vi "Configure Dialog.vi"(8 "error in (no error)":errorcluster, 11 "Initiate Acquisition Msg in":refnum<class "Initiate Acquisition Msg.lvclass">) -> (0 "error out":errorcluster, 2 "Ok?":bool, 3 "Initiate Acquisition Msg out":refnum<class "Initiate Acquisition Msg.lvclass">)   [LabVIEW 2014, in "CS++Scope.lvlib" / "Initiate Acquisition Msg.lvclass"]
uses:
  Initiate Acquisition Msg.lvclass
  Initiate Acquisition Msg.lvclass/Initiate Acquisition Msg.ctl
panel:
  in  "OK Button":bool
  in  "Cancel Button":bool
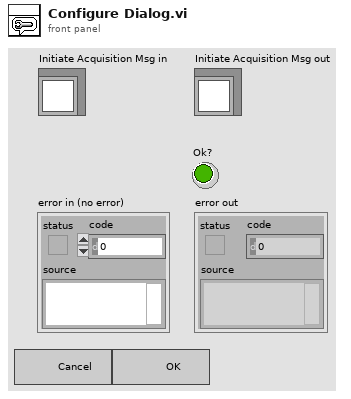
[diagram p1: front panel]
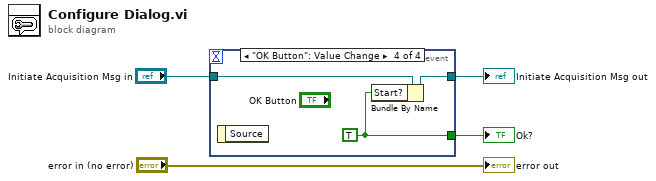
[diagram p0: block diagram]
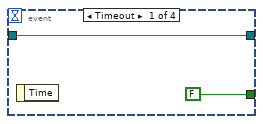
[diagram p2: hidden frame]
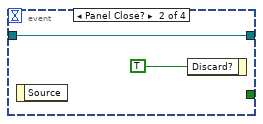
[diagram p3: hidden frame]
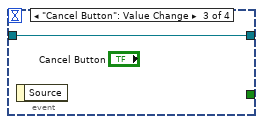
[diagram p4: hidden frame]
diagram:
  n1 = event shown="[3] \"OK Button\": Value Change" {
    selector: _ -> [_ _ _ _]
    dyn-events: _ -> [_ _ _ _]
    timeout: _ -> [_ _ _ _]
    tunnel: [w6 w7 w9 w11] -> w3
    tunnel: "Initiate Acquisition Msg in" -> [w6 w7 w9 w12]
    tunnel: [FALSE _ _ w10] -> w1
    event Timeout {
      n2 = event-data() -> ()  [unwired: 1 in, 1 out]
    }
    event Panel Close? {
      n3 = event-data() -> ()  [unwired: 1 in, 1 out]
      n4 = event-data("Discard?"=TRUE) -> ()  [unwired: 1 in, 1 out]
    }
    event "Cancel Button": Value Change {
      n5 = event-data() -> ()  [unwired: 1 in, 1 out]
    }
    event "OK Button": Value Change {
      w10 = TRUE
      n6 = event-data() -> ()  [unwired: 1 in, 1 out]
      n7 = Bundle By Name(cluster=w12, "Start?"=w10) -> (w11:refnum<class "Initiate Acquisition Msg.lvclass">)
    }
  }
  "Initiate Acquisition Msg out" <- w3
  "Ok?" <- w1
  "error out" <- "error in (no error)"
